vi "Initialize.vi"(8 "error in (no error)":errorcluster, 9 "Spawn Direction":T1, 11 "Base Builder in":refnum<class "Base Builder.lvclass">) -> (0 "error out":errorcluster, 3 "Base Builder out":refnum<class "Base Builder.lvclass">)   [LabVIEW 2015, in "Base Builder.lvclass"]
uses:
  Base Builder.lvclass
  Type Defs/Direction Enum.ctl
  Type Defs/Action Enum.ctl
  Base Builder.lvclass/Base Builder.ctl
  Common/Update Position.vi
  Square/Board Size.vi
  SubVIs/Read-Only Globals.vi
  Type Defs/SB Type Defs.lvlib
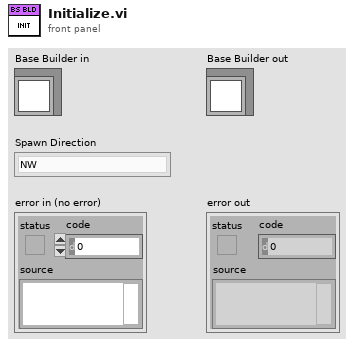
[diagram p1: front panel]
types:
  T1 = typedef "SB Type Defs.lvlib/Direction Enum.ctl" = enum16{"NW", "N", "NE", "E", "SE", "S", "SW", "W"}
  T2 = typedef "SB Type Defs.lvlib/Action Enum.ctl" = enum16{"Wait", "Move", "Attack", "Replicate"}
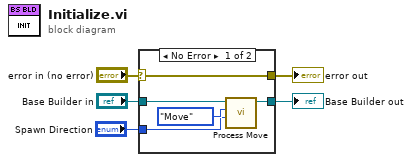
[diagram p0: block diagram]
diagram:
  n1 = case shown="No Error" "error in (no error)" {
    selector: "error in (no error)" -> [w9 w12]
    tunnel: [w9 w12] -> w4
    tunnel: [w8 w11] -> w2
    tunnel: "Base Builder in" -> [w10 w11]
    tunnel: "Spawn Direction" -> [w6 _]
    frame No Error {
      n2 = call "Process Move.vi"("Direction"=w6, "Action"=Action_Enum."Move", "Base Builder In"=w10) -> ("Base Builder Out"=w8:refnum<class "Base Builder.lvclass">)  [unwired: 7 in, 1 out]
    }
    frame Error {
    }
  }
  "error out" <- w4
  "Base Builder out" <- w2
